vi "RecoveryTDMSFile.vi"() -> ()   [LabVIEW 2009]
panel:
  out "error out":errorcluster
  in  "file path (use dialog)":path
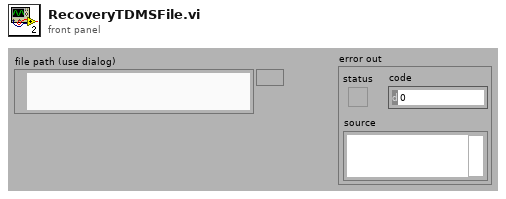
[diagram p1: front panel]
types:
  T1 = enum16{"big-endian, network order", "native, host order", "little-endian"}
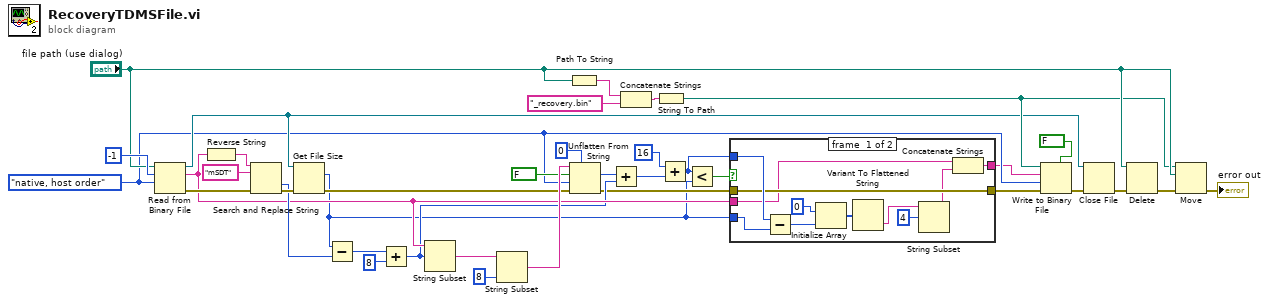
[diagram p0: block diagram]
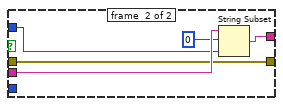
[diagram p2: hidden frame]
diagram:
  w9 = T1."native, host order" ("byte order (0:big-endian, network order)")
  n1 = Read from Binary File(9:w9, 10:-1 ("count (1)"), 11:"file path (use dialog)") -> (0:w34:errorcluster, 2:w22:string, 3:w13:refnum<file>)  [unwired: 3 in, 1 out]
  n2 = Reverse String(1:w22) -> (0:w37:string)
  n3 = Search and Replace String(input string=w37, search string="mSDT", error in=w34) -> (offset past replacement=w33:i32, error out=w35:errorcluster)  [unwired: 5 in, 2 out]
  n4 = Get File Size(file=w13, error in=w35) -> (size (in bytes)=w1:i64, 0:w23:errorcluster)  [unwired: 1 out]
  n5 = Subtract(x=w1, y=w33) -> (x-y=w31:i64)
  n6 = Add(x=w31, y=i64 8) -> (x+y=w10:i64)
  n7 = String Subset(string=w22, offset (0)=w10) -> (substring=w28:string)  [unwired: 1 in]
  n8 = String Subset(string=w28, length (rest)=8 ("length (rest)")) -> (substring=w27:string)  [unwired: 1 in]
  n9 = Path To String(path="file path (use dialog)") -> (string=w18:string)
  n10 = Unflatten From String(type=i64 0, binary string=w27, data includes array or string size? (T)=FALSE, byte order (0:big-endian, network order)=w9, error in (no error)=w23) -> (value=w24:i64, error out=w4:errorcluster)  [unwired: 1 out]
  n11 = Add(x=w24, y=w10) -> (x+y=w7:i64)
  n12 = Concatenate Strings(w18, "_recovery.bin" ("name or relative path")) -> (w16:string)
  n13 = String To Path(string=w16) -> (path=w15:path)
  n14 = Add(x=i64 16, y=w7) -> (x+y=w2:i64)
  n15 = Less?(x=w2, y=w1) -> (x < y?=w5:bool)
  n16 = case shown="True" w5 {
    tunnel: w22 -> [w39 w53]
    tunnel: [w40 w51] -> w6
    tunnel: w4 -> [w41 w50]
    tunnel: [w41 w50] -> w3
    tunnel: w2 -> [w48 w49]
    tunnel: w1 -> [w47 _]
    frame #0 {
      n17 = Subtract(x=w48, y=w47) -> (x-y=w43:i64)
      n18 = Initialize Array(i8 0 ("element"), w43) -> (w46:i8[])
      n19 = Variant To Flattened String(Variant=w46) -> (data string=w45:string)  [unwired: 1 out]
      n20 = String Subset(string=w45, offset (0)=4) -> (substring=w38:string)  [unwired: 1 in]
      n21 = Concatenate Strings(w39, w38) -> (w40:string)
    }
    frame #1 {
      n22 = String Subset(string=w53, offset (0)=0, length (rest)=w49) -> (substring=w51:string)
    }
  }
  n23 = Write to Binary File(file (use dialog)=w15, data=w6, error in=w3, 5:FALSE ("prepend array or string size? (T)"), 9:w9) -> (error out=w14:errorcluster)  [unwired: 1 in, 2 out]
  n24 = Close File(refnum=w13, error in=w14) -> (error out=w12:errorcluster)  [unwired: 1 out]
  n25 = Delete(path (use dialog)="file path (use dialog)", error in=w12) -> (error out=w21:errorcluster)  [unwired: 3 in, 2 out]
  n26 = Move(source path=w15, error in=w21, 10:"file path (use dialog)") -> (error out=→"error out":errorcluster)  [unwired: 2 in, 2 out]
